vi "GSP_SLIT_Global.vi"() -> ()   [LabVIEW 2015]
uses:
  SystemUtil/MotorStates.ctl
  SystemUtil/ThreadStates.ctl
panel:
  out "Slit Hidden?":bool
  in  "Slit Name":string
  in  "Slit Thread State":T1
  in  "Carousel Pos":i32
  in  "Coll Ext Temp":dbl
  in  "Slit Trans State":T2
  in  "Slit Rot State":T2
  in  "SLIT TRANS CPU Temp":dbl
  in  "SLIT ROT CPU Temp":dbl
  out "Slit Online":bool
  in  "Slit#":i32
  in  "Offset to first Position":i32=175
  in  "Counts per Position":dbl=333.0 format="%.2f"
  in  "No Slit Position":i32=1000
  in  "Clear Position":i32=251743
  in  "Detent Position":i32=88865
  in  "Grab Position":i32=285543
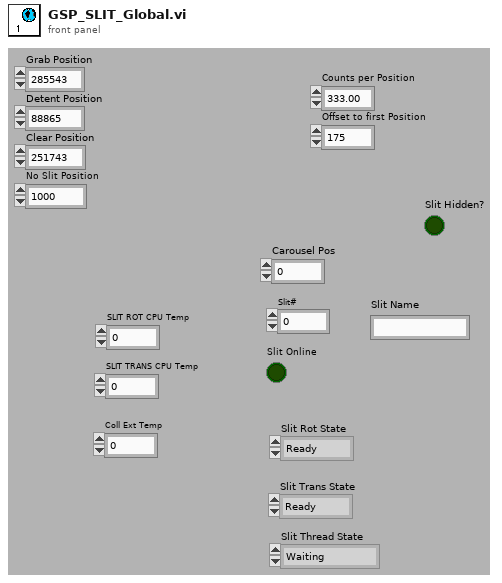
[diagram p1: front panel]
types:
  T1 = typedef "ThreadStates.ctl" = enum16{"Waiting", "Scripting", "Uninitialized", "Error"}
  T2 = typedef "MotorStates.ctl" = enum16{"Ready", "Moving", "Uninitialized", "Error"}
diagram:
